vi "error_popup.vi"(6 "STOP_button_reference":refnum<vi>, 7 "EXIT App If Error? (F)":bool, 8 "error_in":errorcluster) -> (0 "error_out":errorcluster)   [LabVIEW 2020]
uses:
  AULocalize/SubVIs/Get Localized Phrase Compact Interface 0D.vi
  AULocalize/SubVIs/RegisterVI.vi
panel:
  out "Project Title 2":string
  out "Message copy":string
  in  "OK":bool
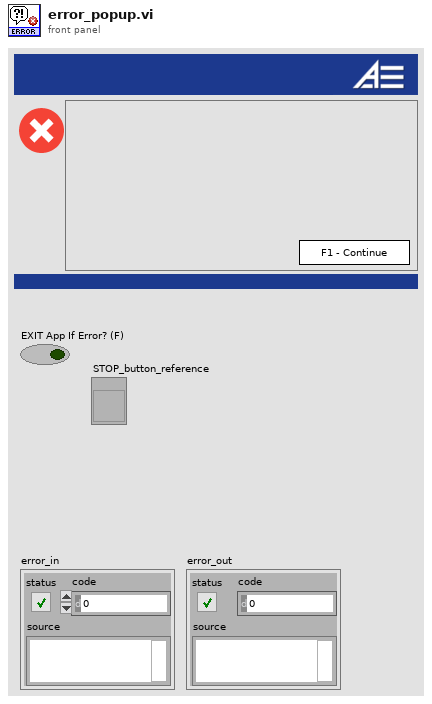
[diagram p1: front panel]
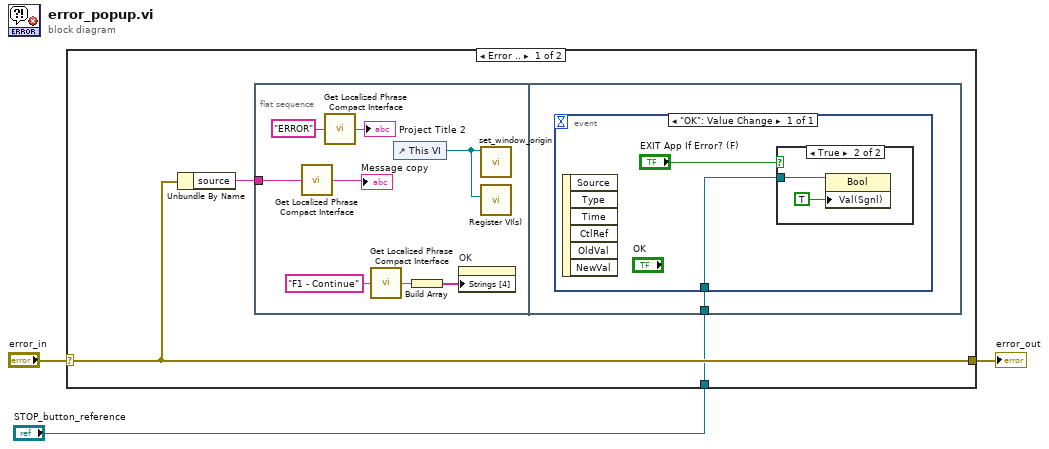
[diagram p0: block diagram]
diagram:
  n1 = case shown="Error .." "error_in" {
    selector: "error_in" -> [w6 w20]
    tunnel: [w6 w20] -> w2
    tunnel: "STOP_button_reference" -> [w4 _]
    frame Error {
      n2 = Unbundle By Name(w6) -> ("source"=w5:string)
      n3 = flat-sequence {
        tunnel: w5 -> [w13]
        tunnel: w4 -> [w15]
        frame #0 {
          n4 = call-poly "Get Localized Phrase Compact Interface.vi"("Key"=w13) -> ("Translated Phrase"=→"Message copy":string)
          n5 = call-poly "Get Localized Phrase Compact Interface.vi"("Key"="ERROR" ("Project Title 2")) -> ("Translated Phrase"=→"Project Title 2":string)
          n6 = call-poly "Get Localized Phrase Compact Interface.vi"("Key"="F1 - Continue") -> ("Translated Phrase"=w9:string)
          n7 = control-ref of="This VI"() -> (w11:refnum<vi>)
          n8 = Build Array(w9) -> (w14:string[])
          n9 = property on="OK" class="Bool"("Strings [4]"=w14) -> ()  [unwired: 2 in, 2 out]
          n10 = call "set_window_origin.vi"("this_vi_reference"=w11) -> ()  [unwired: 10 in, 1 out]
          n11 = call-poly "Register VI(s).vi"("VI Ref"=w11) -> ()  [unwired: 9 in, 2 out]
        }
        frame #1 {
          n12 = event shown="[0] \"OK\": Value Change" {
            selector: _ -> [_]
            dyn-events: _ -> [_]
            timeout: _ -> [_]
            tunnel: w15 -> [w17]
            event "OK": Value Change {
              n13 = event-data() -> ()  [unwired: 1 in, 6 out]
              n14 = case shown="True" "EXIT App If Error? (F)" {
                tunnel: w17 -> [_ w19]
                frame False {
                }
                frame True {
                  n15 = property on="Property Node" class="Bool"(reference=w19, "Val(Sgnl)"=TRUE ("Value (Signaling)")) -> ()  [unwired: 1 in, 2 out]
                }
              }
            }
          }
        }
      }
    }
    frame No Error {
    }
  }
  "error_out" <- w2
